vi "hosts.deserialize.orderbook.entries.vi"(11 "DataIn":u64[](array[numeric])) -> (3 "OrderBook.Entries":T1[](array[typedef]))   [LabVIEW 2020]
uses:
  arty/application/orderbook.entry.ctl
  arty/application/orderbook.result.type.ctl
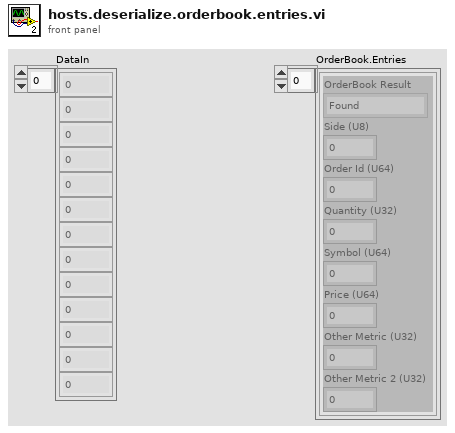
[diagram p1: front panel]
types:
  T1 = typedef "orderbook.entry.ctl" = cluster{"OrderBook Result":T2, "Side (U8)":u8, "Order Id (U64)":u64, "Quantity (U32)":u32, "Symbol (U64)":u64, "Price (U64)":u64, "Other Metric (U32)":u32, "Other Metric 2 (U32)":u32}
  T2 = typedef "orderbook.result.type.ctl" = enum16{"Found", "Not.Found"}
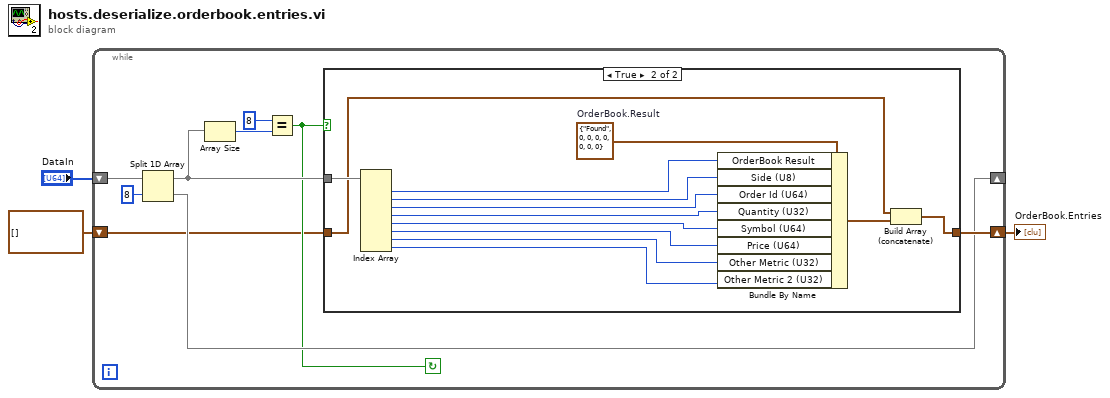
[diagram p0: block diagram]
diagram:
  n1 = while {
    shift-right: [w8] -> _
    shift-left: "DataIn" -> [w12]
    shift-right: [w10] -> w1
    shift-left: T1[] [] -> [w4]
    stop <- w5 continue-if-true
    n2 = Split 1D Array(array=w12, index=8) -> (first subarray=w9:u64[], second subarray=w8:u64[])
    n3 = Array Size(array=w9) -> (size(s)=w7:i32)
    n4 = Equal?(x=8, y=w7) -> (x = y?=w5:bool)
    n5 = case shown="True" w5 {
      tunnel: [w13 w16] -> w10
      tunnel: w9 -> [_ w18]
      tunnel: w4 -> [w13 w15]
      frame False {
      }
      frame True {
        w14 = T1 {"OrderBook Result"=enum."Found", "Side (U8)"=0, "Order Id (U64)"=0, "Quantity (U32)"=0, "Symbol (U64)"=0, "Price (U64)"=0, "Other Metric (U32)"=0, "Other Metric 2 (U32)"=0}  # OrderBook.Result
        n6 = Index Array(array=w18) -> (element #1=w26:u64, element #2=w25:u64, element #3=w24:u64, element #4=w23:u64, element #5=w22:u64, element #6=w21:u64, element #7=w20:u64, element #8=w19:u64)  [unwired: 8 in]
        n7 = Bundle By Name(cluster=w14, "OrderBook Result"=w26, "Side (U8)"=w25, "Order Id (U64)"=w24, "Quantity (U32)"=w23, "Symbol (U64)"=w22, "Price (U64)"=w21, "Other Metric (U32)"=w20, "Other Metric 2 (U32)"=w19) -> (w17:T1)
        n8 = Build Array (concatenate)(w15, w17) -> (w16:T1[])
      }
    }
  }
  "OrderBook.Entries" <- w1
